vi "PC_Pub_imgFile updAppImgInfo.vi"(8 "error in (no error)":errorcluster, 10 "RTCtrlrPath":path, 11 "imgFile in":refnum<class "PC_Pub_imgFile.lvclass">) -> (0 "error out":errorcluster, 3 "imgFile out":refnum<class "PC_Pub_imgFile.lvclass">)   [LabVIEW 2018, in "PC_Pub_imgFile.lvclass"]
uses:
  PC_Pub_imgFile.lvclass
  PC_Pub_imgFile.lvclass/PC_Pub_imgFile.ctl
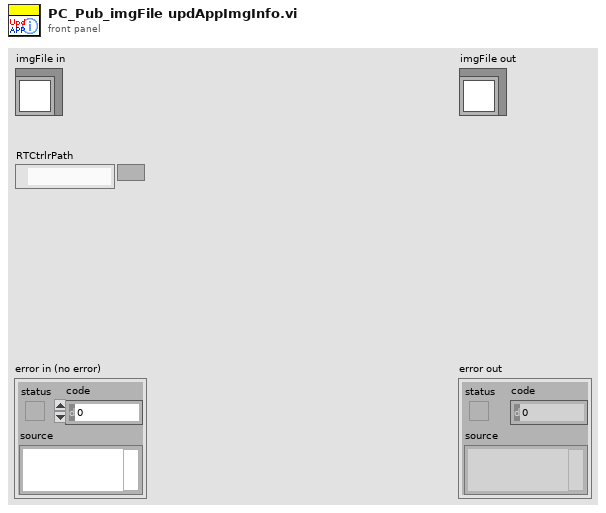
[diagram p1: front panel]
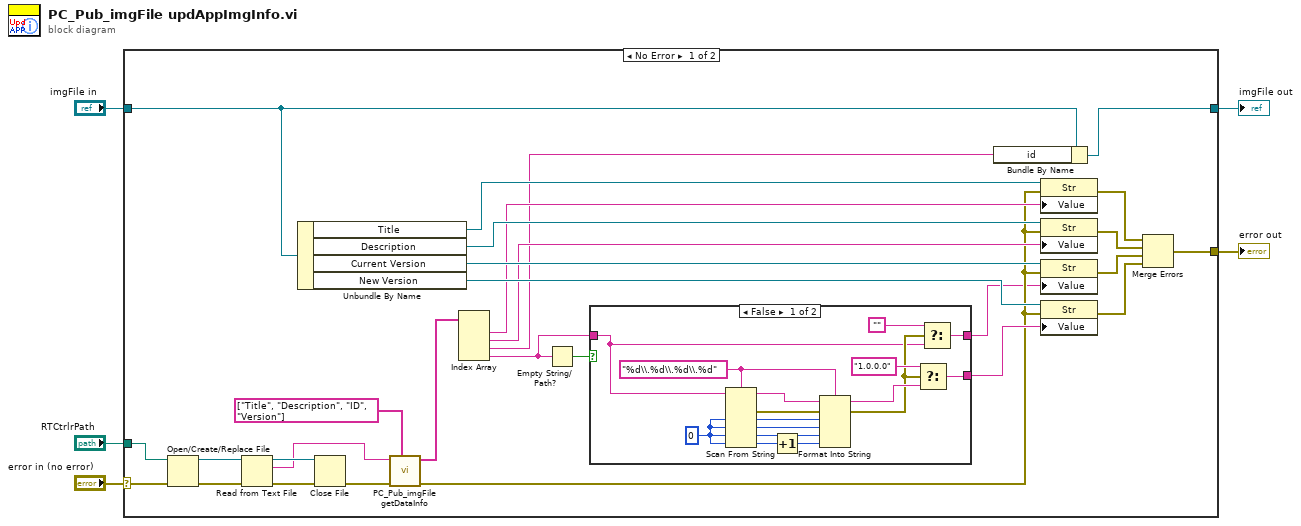
[diagram p0: block diagram]
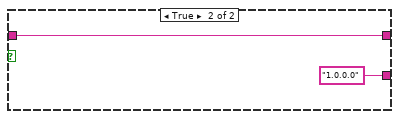
[diagram p2: hidden frame]
diagram:
  n1 = case shown="No Error" "error in (no error)" {
    selector: "error in (no error)" -> [w29 w54]
    tunnel: [w11 w54] -> w4
    tunnel: [w7 w53] -> w2
    tunnel: "imgFile in" -> [w8 w53]
    tunnel: "RTCtrlrPath" -> [w30 _]
    frame No Error {
      n2 = Open/Create/Replace File(file path (use dialog)=w30, error in=w29) -> (refnum out=w34:refnum<file>, error out=w33:errorcluster)  [unwired: 4 in, 1 out]
      n3 = Read from Text File(file (use dialog)=w34, error in=w33) -> (refnum out=w32:refnum<file>, text=w28:string, error out=w31:errorcluster)  [unwired: 2 in, 1 out]
      n4 = Unbundle By Name(w8) -> ("Title"=w24:refnum<vi>, "Description"=w23:refnum<vi>, "Current Version"=w22:refnum<vi>, "New Version"=w21:refnum<vi>)
      n5 = Close File(refnum=w32, error in=w31) -> (error out=w27:errorcluster)  [unwired: 1 out]
      n6 = call "PC_Pub_imgFile getDataInfo.vi"("getTitle"=string[] ["Title", "Description", "ID", "Version"], "error in (no error)"=w27, "dataString"=w28) -> ("error out"=w16:errorcluster, "getValue"=w25:string[])  [unwired: 7 in]
      n7 = Index Array(array=w25) -> (element #1=w20:string, element #2=w19:string, element #3=w6:string, element #4=w9:string)  [unwired: 4 in]
      n8 = Empty String/Path?(string/path=w9) -> (empty?=w18:bool)
      n9 = case shown="False" w18 {
        tunnel: [w39 "1.0.0.0"] -> w17
        tunnel: w9 -> [w35 w51]
        tunnel: [w38 w51] -> w10
        frame False {
          w50 = u16 0
          w46 = "%d\\.%d\\.%d\\.%d" ("format string")
          n10 = Scan From String(format string=w46, input string=w35, default 1=w50, default 2=w50, default 3=w50, default 4=w50) -> (remaining string=w47:string, error out=w41:errorcluster, output 1=w45:u16, output 2=w44:u16, output 3=w43:u16, output 4=w48:u16)  [unwired: 2 in, 1 out]
          n11 = Increment(x=w48) -> (x+1=w42:u16)
          n12 = Format Into String(format string=w46, initial string=w47, error in=w41, w45, w44, w43, w42) -> (resulting string=w40:string, error out=w36:errorcluster)
          n13 = Select(t="1.0.0.0", s=w36, f=w40) -> (s? t:f=w39:string)
          n14 = Select(t="", s=w36, f=w35) -> (s? t:f=w38:string)
        }
        frame True {
        }
      }
      n15 = Bundle By Name(cluster=w8, "id"=w6) -> (w7:refnum<class "PC_Pub_imgFile.lvclass">)
      n16 = property class="Str"(reference=w24, error in=w16, "Value"=w20) -> (error out=w15:errorcluster)  [unwired: 1 out]
      n17 = property class="Str"(reference=w23, error in=w16, "Value"=w19) -> (error out=w14:errorcluster)  [unwired: 1 out]
      n18 = property class="Str"(reference=w22, error in=w16, "Value"=w10) -> (error out=w13:errorcluster)  [unwired: 1 out]
      n19 = property class="Str"(reference=w21, error in=w16, "Value"=w17) -> (error out=w12:errorcluster)  [unwired: 1 out]
      n20 = Merge Errors(w15, w14, w13, w12) -> (w11:errorcluster)
    }
    frame Error {
    }
  }
  "error out" <- w4
  "imgFile out" <- w2
